vi "List Tables.vi"(8 "Error In":errorcluster) -> (0 "Error Out":errorcluster, 3 "Tables":string[](array[string]))   [LabVIEW 2018, in "Database.lvlib"]
uses:
  Database.lvlib
  Action.ctl
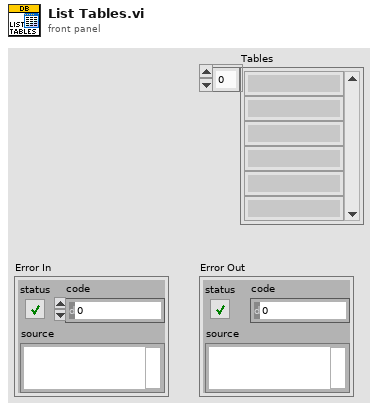
[diagram p1: front panel]
types:
  T1 = typedef "Database.lvlib/Action.ctl" = enum16{"Init", "List Tables", "List Columns", "Query", "Close"}
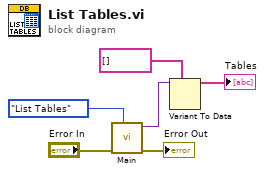
[diagram p0: block diagram]
diagram:
  n1 = call "Main.vi"("Action"=Action."List Tables", "Error In"="Error In") -> ("Error Out"=→"Error Out":errorcluster, "Output"=w4:variant)  [unwired: 8 in]
  n2 = Variant To Data(type=string[] [], Variant=w4) -> (data=→"Tables":string[])  [unwired: 1 in, 1 out]
